vi "replaceConditionToken.vi"(8 "error in (no error)":errorcluster, 10 "Query In":string, 11 "Credit Transactions in":refnum<class "CreditTransactionList.lvclass">) -> (0 "error out":errorcluster, 2 "Query Out":string, 3 "Credit Transactions out":refnum<class "CreditTransactionList.lvclass">)   [LabVIEW 2018, in "CreditTransactionList.lvclass"]
uses:
  CreditTransactionList.lvclass
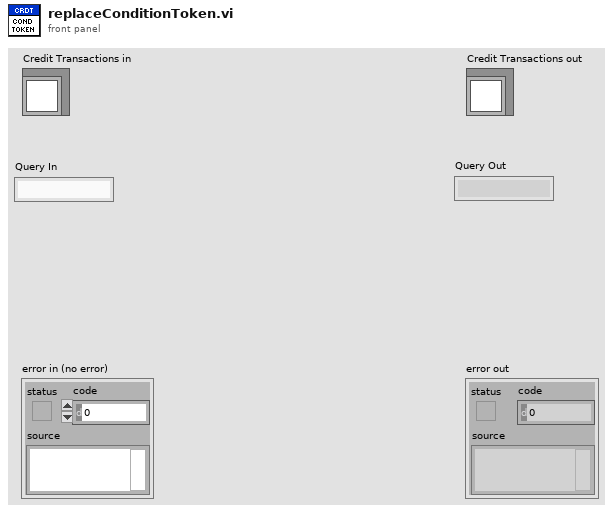
[diagram p1: front panel]
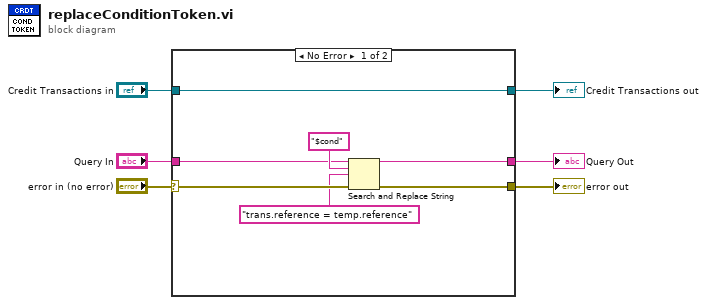
[diagram p0: block diagram]
diagram:
  n1 = case shown="No Error" "error in (no error)" {
    selector: "error in (no error)" -> [w8 w15]
    tunnel: [w10 w16] -> w2
    tunnel: "Query In" -> [w9 w14]
    tunnel: "Credit Transactions in" -> [w10 w16]
    tunnel: [w13 w15] -> w3
    tunnel: [w12 w14] -> w1
    frame No Error {
      n2 = Search and Replace String(input string=w9, search string="$cond", replace string="trans.reference = temp.reference", error in=w8) -> (result string=w12:string, error out=w13:errorcluster)  [unwired: 4 in, 2 out]
    }
    frame Error {
    }
  }
  "error out" <- w3
  "Credit Transactions out" <- w2
  "Query Out" <- w1
